vi "Launch_Component.vi"() -> ()   [LabVIEW 2022 SP3]
uses:
  Components/ViPER.lvlibp/ViPER.lvclass
panel:
  in  "Config XML":string="<?xml version=\"1.0\" encoding=\"UTF-8\" standalone=\"no\" ?>\n<Object>\n\n  <Name>Count</Name>\n\n  <Class>Frequency_Counter_BK</Class>\n\n  <Config>\n    <NumElts>3</NumElts>\n    <Refnum>\n      <Name>ComPort</Name>\n      <RefKind>VISA</RefKind>\n      <Val/>\n</Refnum>\n    <I8>\n      <Name>Function</Name>\n      <Val>0</Val>\n</I8>\n    <I8>\n      <Name>Gate_Time</Name>\n      <Val>0</Val>\n</I8>\n</Config>  <Ancestors>\n    <Ancestor>\n      <Class>Frequency_Counter_Base</Class>\n      <Config>\n        <NumElts>1</NumElts>\n        <String>\n          <Name>default</Name>\n          <Val/>\n</String>\n</Config>    </Ancestor>\n  </Ancestors>\n\n</Object>\n"
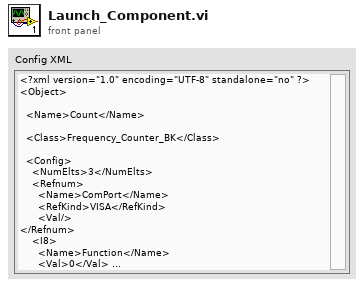
[diagram p1: front panel]
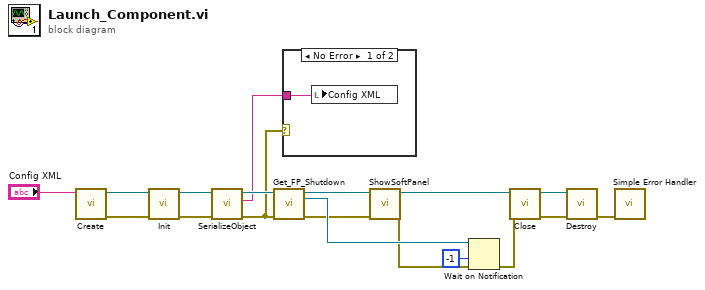
[diagram p0: block diagram]
diagram:
  n1 = call "Create.vi"("Config XML"="Config XML") -> ("error out"=w14:errorcluster, "reference out"=w15:refnum<class "ViPER.lvclass">)  [unwired: 9 in]
  n2 = call-dynamic "Init.vi"("error in (no error)"=w14, "reference in"=w15) -> ("error out"=w5:errorcluster, "reference out"=w4:refnum<class "ViPER.lvclass">)  [unwired: 8 in]
  n3 = call-dynamic "SerializeObject.vi"("error in (no error)"=w5, "ViPER_Base in"=w4) -> ("error out"=w1:errorcluster, "Object XML"=w2:string, "ViPER_Base out"=w3:refnum<class "ViPER.lvclass">)  [unwired: 7 in]
  n4 = call "Get_FP_Shutdown.vi"("ViPER_Base in"=w3, "error in (no error)"=w1) -> ("ViPER_Base out"=w12:refnum<class "ViPER.lvclass">, "SoftFP_Shutdown"=w13:refnum<notifier>, "error out"=w11:errorcluster)  [unwired: 10 in, 1 out]
  n5 = case shown="No Error" w1 {
    tunnel: w2 -> [w19 _]
    frame No Error {
      n6 = local write "Config XML"(w19) -> ()
    }
    frame Error {
    }
  }
  n7 = call-dynamic "ShowSoftPanel.vi"("error in (no error)"=w11, "Driver in"=w12) -> ("error out"=w10:errorcluster, "Driver out"=w9:refnum<class "ViPER.lvclass">)  [unwired: 7 in, 1 out]
  n8 = Wait on Notification(notifier=w13, timeout in ms (-1)=-1, error in (no error)=w10) -> (error out=w18:errorcluster)  [unwired: 1 in, 3 out]
  n9 = call-dynamic "Close.vi"("error in (no error)"=w18, "reference in"=w9) -> ("error out"=w8:errorcluster, "reference out"=w6:refnum<class "ViPER.lvclass">)  [unwired: 8 in]
  n10 = call "Destroy.vi"("error in (no error)"=w8, "reference in"=w6) -> ("error out"=w7:errorcluster)  [unwired: 9 in]
  n11 = call <vilib>:"Simple Error Handler.vi"("error in (no error)"=w7) -> ()  [unwired: 4 in, 5 out]
